vi "2D_data.vi"(0 "String":string) -> (1 "Error detected!":bool, 2 "output array":string[][](array[string]))   [LabVIEW 2012]
panel:
  # "-1) Error! unknown command detected"
  # "0) //comment that start with double forward slash"
  # "1) LINE<space>[Displacement]<space>[Speed]<space>[Current]"
  # "2) JUMP<space>[Displacement]<space>[Speed]"
  # "3) ARC<space>[Type]<space>[Radius]<space>[Current]"
  # "4) LINE1<space>[Displacement]<space>[Speed]<space>[Current]<space>[wait]<space>[repetitions]"
  # "5) LINE2<space>[Displacement]<space>[Speed]<space>[Current]<space>[t_before]<space>[frequency]<space>[Amplitude]<space>[t_enable]"
  # "6) WAIT<space>[Time]"
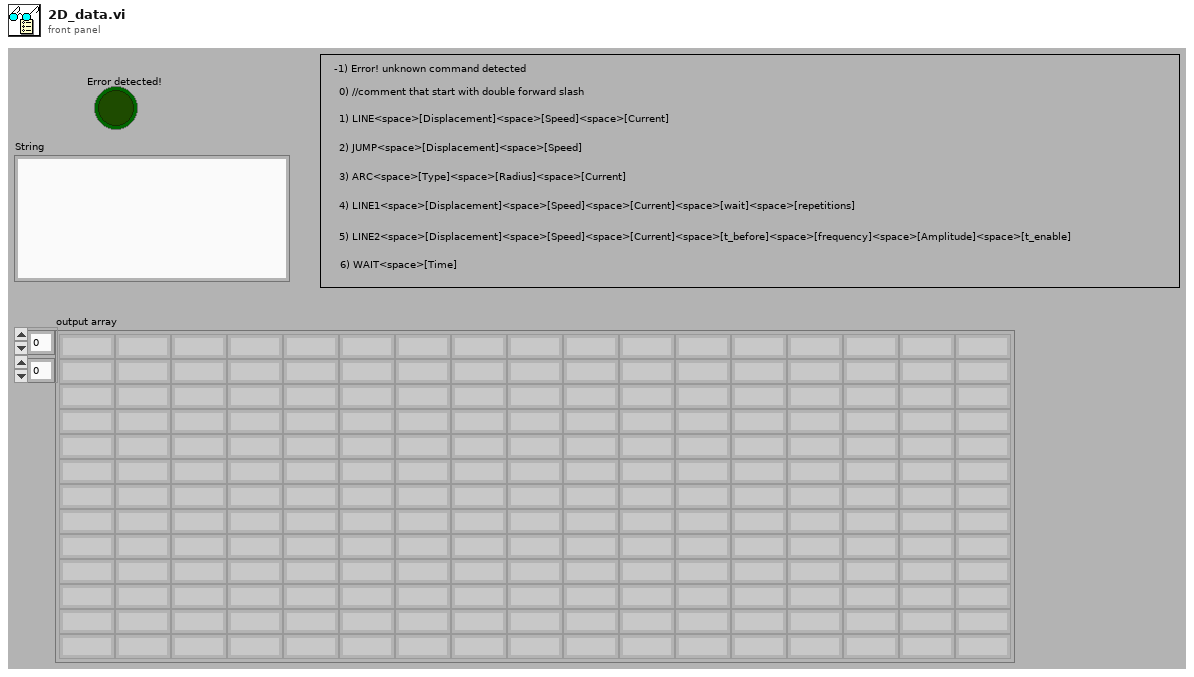
[diagram p1: front panel]
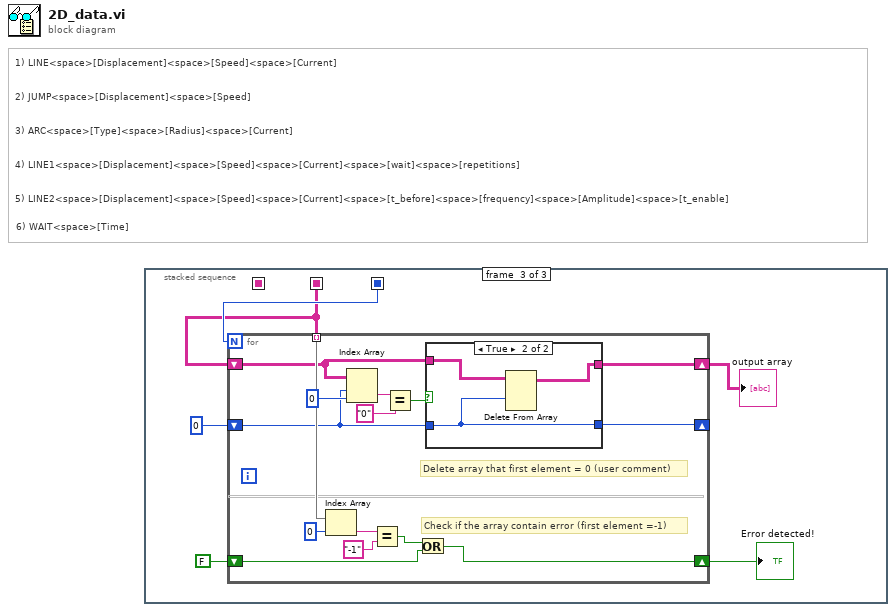
[diagram p0: block diagram]
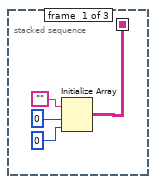
[diagram p2: hidden frame]
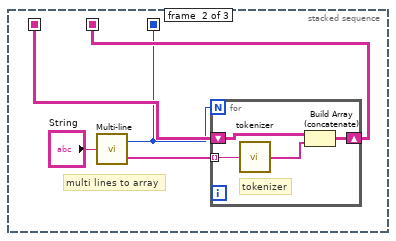
[diagram p3: hidden frame]
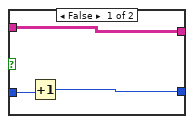
[diagram p4: hidden frame]
diagram:
  # "6) WAIT<space>[Time]"
  # "5) LINE2<space>[Displacement]<space>[Speed]<space>[Current]<space>[t_before]<space>[frequency]<space>[Amplitude]<space>[t_enable]"
  # "4) LINE1<space>[Displacement]<space>[Speed]<space>[Current]<space>[wait]<space>[repetitions]"
  # "3) ARC<space>[Type]<space>[Radius]<space>[Current]"
  # "2) JUMP<space>[Displacement]<space>[Speed]"
  # "1) LINE<space>[Displacement]<space>[Speed]<space>[Current]"
  n1 = stacked-sequence {
    seq-local: [w1 _ _] -> [_ w7 _]
    seq-local: [_ w6 _] -> [_ _ w16]
    seq-local: [_ w5 _] -> [_ _ w19]
    frame #0 {
      n2 = Initialize Array("", 0 ("dimension size"), 0 ("dimension size")) -> (w1:string[][])
    }
    frame #1 {
      # "multi lines to array"
      n3 = call "Multi-line.vi"("String"="String") -> ("Array"=w8:string[], "Array size"=w5:i32)
      n4 = for {
        N: w5 -> [_]
        tunnel: w8 -> [w13] mode=indexing
        shift-right: [w10] -> w6
        shift-left: w7 -> [w11]
        # "tokenizer"
        n5 = call "tokenizer.vi"("Input String"=w13) -> ("Output Array"=w12:string[])
        n6 = Build Array (concatenate)(w11, w12) -> (w10:string[][])
      }
    }
    frame #2 {
      n7 = for {
        N: w19 -> [_]
        tunnel: w16 -> [w34] mode=indexing
        shift-right: [w29] -> w18
        shift-left: FALSE -> [w28]
        shift-right: [w23] -> w15
        shift-left: w16 -> [w22]
        shift-right: [w20] -> _
        shift-left: u16 0 -> [w21]
        # "Delete array that first element = 0 (user comment)"
        # "Check if the array contain error (first element =-1)"
        n8 = Index Array(array=w34, index=0) -> (element=w32:string)
        n9 = Index Array(array=w22, index (row)=w21, index (col)=0 ("disabled index (col)")) -> (element=w27:string)
        n10 = Equal?(x=w32, y="-1") -> (x = y?=w30:bool)
        n11 = Equal?(x=w27, y="0") -> (x = y?=w25:bool)
        n12 = Or(x=w30, y=w28) -> (x .or. y?=w29:bool)
        n13 = case shown="True" w25 {
          tunnel: w22 -> [w37 w40]
          tunnel: w21 -> [w36 w38]
          tunnel: [w37 w39] -> w23
          tunnel: [w35 w38] -> w20
          frame False {
            n14 = Increment(x=w36) -> (x+1=w35:u16)
          }
          frame True {
            n15 = Delete From Array(array=w40, index (row)=w38) -> (array with subset deleted=w39:string[][])  [unwired: 2 in, 1 out]
          }
        }
      }
      "Error detected!" <- w18
      "output array" <- w15
    }
  }
